vi "Render True Section.vi"(8 "Error In":errorcluster) -> (0 "Error Out":errorcluster)   [LabVIEW 2018, in "Tests.lvlib" / "Render.lvlib"]
uses:
  Render.lvlib
  <vilib>/addons/_JKI Toolkits/Caraya/classes/Test/Test.lvclass
  <vilib>/addons/_JKI Toolkits/Caraya/classes/Assert/Assert.lvclass
  src/Toolkit/Toolkit.lvlib
  src/Toolkit/Data/Map/Map.lvclass
  src/Toolkit/Low-Level/Support/Lex String.vi
  src/Toolkit/Data/Map/Support/From Datum.vi
  src/Toolkit/Data/Boolean/Boolean.lvclass
  src/Toolkit/Low-Level/Support/Render to String.vi
  src/Toolkit/Low-Level/Context/Compiler.lvclass
  D:/Users/cfield/Code/Field R&D Services/Labstache/src/Toolkit/Data/Datum/Datum.lvclass
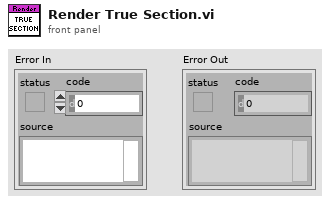
[diagram p1: front panel]
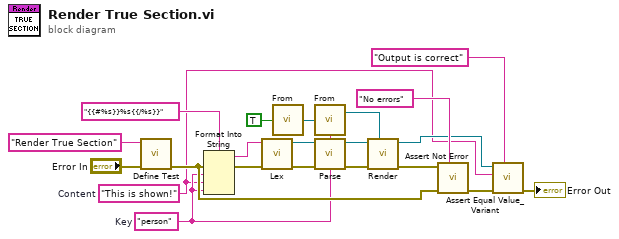
[diagram p0: block diagram]
diagram:
  w2 = "This is shown!"  # Content
  w3 = "person"  # Key
  n1 = call <vilib>:"Define Test.vi"("error in (no error)"="Error In", "Label (VI Title)"="Render True Section") -> ("error out"=w9:errorcluster)  [unwired: 9 in]
  n2 = Format Into String(format string="{{#%s}}%s{{/%s}}", error in=w9, w3, w2, w3) -> (resulting string=w6:string, error out=w8:errorcluster)  [unwired: 1 in]
  n3 = call-poly "Lex.vi"("Error In"=w8, "Context In"=w6) -> ("Error Out"=w11:errorcluster, "Context Out"=w12:refnum<class "Compiler.lvclass">)  [unwired: 7 in, 1 out]
  n4 = call "From.vi"("Value"=TRUE) -> ("Boolean"=w4:refnum<class "Boolean.lvclass">)
  n5 = call-poly "From.vi"("Value"=w4, "Key"=w3) -> ("Map"=w10:refnum<class "Map.lvclass">)
  n6 = call "Parse.vi"("Error In"=w11, "Context In"=w12) -> ("Error Out"=w13:errorcluster, "Context Out"=w1:refnum<class "Compiler.lvclass">)  [unwired: 7 in, 1 out]
  n7 = call-poly "Render.vi"(7:w10, "Error In"=w13, "Context In"=w1) -> ("Error Out"=w15:errorcluster, "Context Out"=w14:refnum<class "Compiler.lvclass">)  [unwired: 6 in, 1 out]
  n8 = call <vilib>:"Assert Not Error.vi"("Label"="No errors", "error in (no error)"=w9, "Not Error?"=w15) -> ("error out"=w18:errorcluster)  [unwired: 8 in]
  n9 = call <vilib>:"Assert Equal Value_Variant.vi"("Label"="Output is correct", "error in (no error)"=w18, "Y"=w2, "X"=w14) -> ("error out"=→"Error Out":errorcluster)  [unwired: 7 in]
